vi "ATS_ErrorCode.vi"(6 "Message":string, 7 "ErrorCode":u32) -> (3 "error out":errorcluster)   [LabVIEW 2015]
doc: "_____AlazarTech, Scope_____\n\nInterpretation of the ErrorCode.\n\nErrorCode:\n0: no error\n511: No board found \n512: no error\n512++: see list of API error code"
uses:
  ATSApi.dll
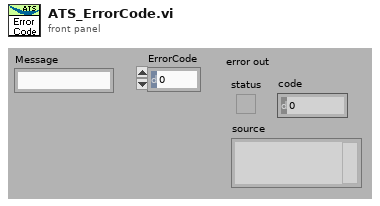
[diagram p1: front panel]
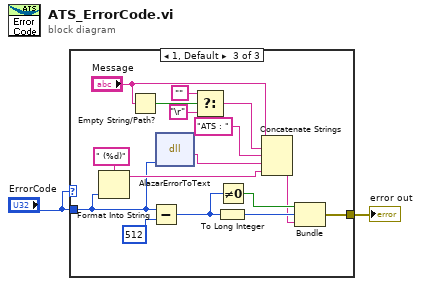
[diagram p0: block diagram]
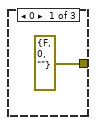
[diagram p2: hidden frame]
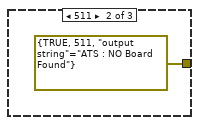
[diagram p3: hidden frame]
diagram:
  n1 = case shown="1, Default" "ErrorCode" {
    tunnel: "ErrorCode" -> [_ _ w5]
    tunnel: [cluster{bool, i32, "output string":string} {FALSE, 0, "output string"=""} cluster{bool, i32, "output string":string} {TRUE, 511, "output string"="ATS : NO Board Found"} w19] -> w2
    frame 0 {
    }
    frame 511 {
    }
    frame 1, Default {
      n2 = Format Into String(format string=" (%d)", w5) -> (resulting string=w8:string)  [unwired: 2 in, 1 out]
      n3 = Empty String/Path?(string/path="Message") -> (empty?=w13:bool)
      n4 = Subtract(x=w5, y=u32 512) -> (x-y=w17:u32)
      n5 = dll-call lib="C:/IntensityOCT/trunk/ATSApi.dll" fn="AlazarErrorToText"("ErrorCode"=w5) -> (w6:string)  [unwired: 4 in, 2 out]
      n6 = Select(t="", s=w13, f="\r") -> (s? t:f=w12:string)
      n7 = To Long Integer(number=w17) -> (32bit integer=w16:i32)
      n8 = Not Equal To 0?(x=w17) -> (x != 0?=w18:bool)
      n9 = Concatenate Strings("Message", w12, "ATS : " ("string (\"\")"), w6, w8) -> (w15:string)
      n10 = Bundle(w18, w16, w15) -> (w19:errorcluster)  [unwired: 1 in]
    }
  }
  "error out" <- w2
